vi "LoadSubvi.vi"(2 "State In 2":T1, 3 "path":path) -> (0 "Reply":string[](array[string]), 1 "State In":T1)   [LabVIEW 2018, in "ConPane Wrapper.xnode"]
uses:
  ConPane Wrapper.xnode
  State.ctl
  <vilib>/picture/picture.llb/imagedata.ctl
  <vilib>/XNodeSupport/XNodeTerm3Array.ctl
  <vilib>/XNodeSupport/XNodeTerm3.ctl
  <vilib>/XNodeSupport/XNodeString.ctl
  <vilib>/XNodeSupport/XNodeVariant.ctl
  <vilib>/XNodeSupport/XNodeRect32.ctl
  <vilib>/XNodeSupport/XNodeInt.ctl
  <vilib>/XNodeSupport/XNodeBool.ctl
  <vilib>/XNodeSupport/XNodeTermDirection.ctl
  Term Types.ctl
  Term Type.ctl
  <userlib>/_LAVAcr/Scripting Tools/XNode Support/XNode Support.lvlib
  <vilib>/XNodeSupport/NI_XNodeSupport.lvlib
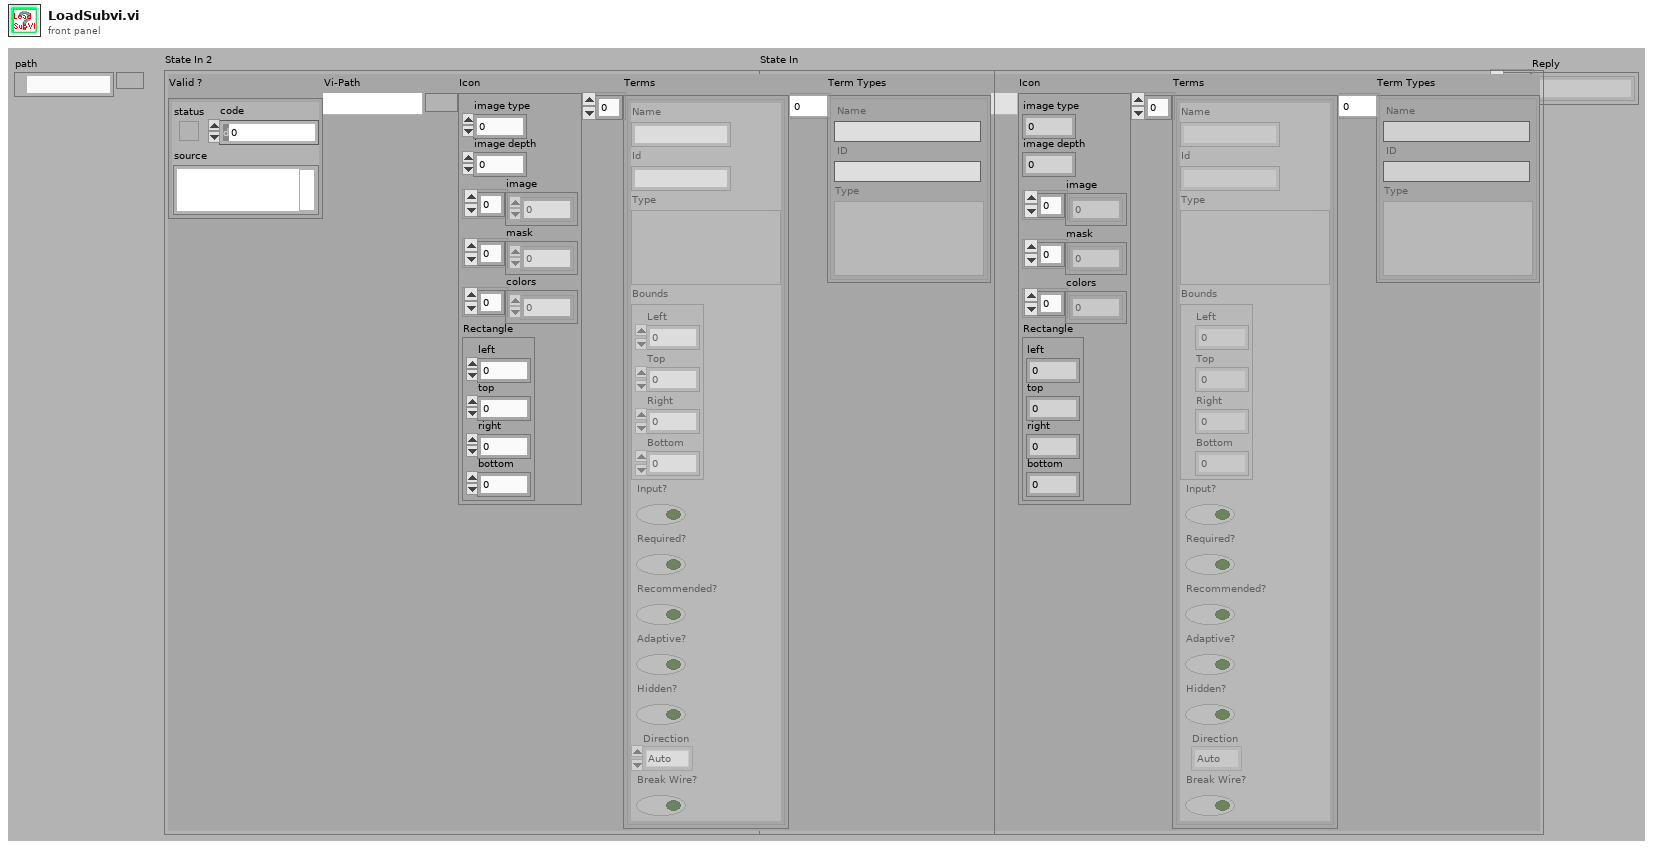
[diagram p1: front panel]
types:
  T1 = typedef "ConPane Wrapper.xnode/State.ctl" = cluster{"Valid ?":errorcluster, "Vi-Path":path, "Icon":T2, "Terms":T3, "Term Types":T11}
  T2 = typedef "imagedata.ctl" = cluster{"image type":i32, "image depth":i32, "image":u8[], "mask":u8[], "colors":u32[], "Rectangle":cluster{"left":i16, "top":i16, "right":i16, "bottom":i16}}
  T3 = typedef "NI_XNodeSupport.lvlib/XNodeTerm3Array.ctl" = T4[]
  T4 = typedef "NI_XNodeSupport.lvlib/XNodeTerm3.ctl" = cluster{"Name":T5, "Id":T5, "Type":T6, "Bounds":T7, "Input?":T9, "Required?":T9, "Recommended?":T9, "Adaptive?":T9, "Hidden?":T9, "Direction":T10, "Break Wire?":T9}
  T5 = typedef "NI_XNodeSupport.lvlib/XNodeString.ctl" = string
  T6 = typedef "NI_XNodeSupport.lvlib/XNodeVariant.ctl" = variant
  T7 = typedef "NI_XNodeSupport.lvlib/XNodeRect32.ctl" = cluster{"Left":T8, "Top":T8, "Right":T8, "Bottom":T8}
  T8 = typedef "NI_XNodeSupport.lvlib/XNodeInt.ctl" = i32
  T9 = typedef "NI_XNodeSupport.lvlib/XNodeBool.ctl" = bool
  T10 = typedef "NI_XNodeSupport.lvlib/XNodeTermDirection.ctl" = enum32{"Auto", "Up", "Down", "Left", "Right", "Center"}
  T11 = typedef "Term Types.ctl" = T12[]
  T12 = typedef "Term Type.ctl" = cluster{"Name":string, "ID":string, "Type":variant}
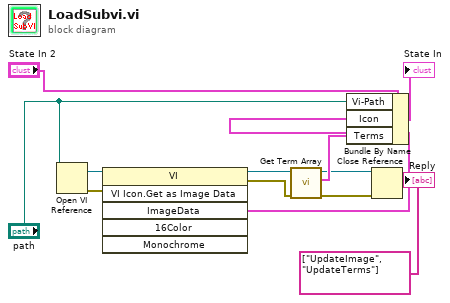
[diagram p0: block diagram]
diagram:
  n1 = Open VI Reference(vi path="path") -> (vi reference=w6:refnum<vi>, error out=w5:errorcluster)  [unwired: 2 in, 3 out]
  n2 = invoke class="VI" method="VI Icon.Get as Image Data"(reference=w6, error in=w5) -> (reference out=w8:refnum<vi>, error out=w9:errorcluster, "ImageData"=w7:T2)  [unwired: 4 in, 3 out]
  n3 = call <userlib>:"Get Term Array.vi"("error in (no error)"=w9, "VI Refnum"=w8) -> ("error out"=w10:errorcluster, "Terminals Array"=w12:T4[], "VI Reference out"=w11:refnum<vi>)  [unwired: 7 out]
  n4 = Bundle By Name(cluster="State In 2", "Vi-Path"="path", "Icon"=w7, "Terms"=w12) -> (→"State In":T1)
  n5 = Close Reference(reference=w11, error in (no error)=w10) -> ()  [unwired: 1 out]
  "Reply" <- string[] ["UpdateImage", "UpdateTerms"] ("Reply")
